vi "State Estimator.vi"(0 "Error In":errorcluster, 1 "State Estimate In":refnum<data-value>, 5 "Matrix":T2, 7 "Configuration":T1={"Accelerometer Bias"={"X (m/s)"=0.0, "Y (m/s)"=0.0, "Z (m/s)"=0.0}, "Gyroscope Bias"={"X (m/s)"=0.0, "Y (m/s)"=0.0, "Z (m/s)"=0.0}, "Steering Motor Gear Ratio"=111.0, "Steering Pully Gear Ratio"=1.0, "Steering Encoder CPR"=500.0, "Steering Motor Max RPM"=4000.0, "Wheelbase (m)"=1.12, "Fork Angle (rad)"=1.3, "Balancing Controller"={"Kp (/s)"=1.3, "Kd (1)"=3.0}, "Max Allowed Steering Angle (rad)"=0.7, "Task Periods"={"Emergency Stop (us)"=10000, "IMU (us)"=10000, "Steering Motor Encoder (us)"=10000, "State Estimator (us)"=10000, "Balancing Controller (us)"=10000, "GNSS (us)"=10000, "Logging (us)"=50000, "Drive Motor (us)"=100000, "Visualization (us)"=100000}, "Drive Motor Gear Ratio"=250.0, "lr"=0.4964, "lf"=0.5986, "lambda"=1.2217, "k1"=0.004472, "k2"=0.09678, "e1_max"=11.331, "Ad_t"=0.95971, "Bd_t"=0.01, "C_t"=2.20588, "D_t"=0.0, "Wheel radius"=0.311}, 9 "Iteration":dbl, 11 "Measurement In":refnum<data-value>, 12 "Balancing controller In":refnum<data-value>) -> (4 "Error out":errorcluster, 15 "Measurement Out":refnum<data-value>)   [LabVIEW 2021]
uses:
  Measurements.ctl
  IMU/IMU Data.ctl
  Steering Motor Encoder/Steering Motor Encoder Data.ctl
  GNSS/GNSS Data.ctl
  Logging/Controller Data.ctl
  Drive Motor/Drive Motor Data.ctl
  Steering Motor/Steering Motor Data.ctl
  State Estimate.ctl
  Configuration/Configuration.ctl
panel:
  out "Flag GPS":dbl
  out "State Estimate Out":refnum<data-value>
  out "data value":T3
  out "output cluster":T6 {"Y (m)" format="%#_10g"; "X (m)" format="%#_10g"}
  out "Balancing controller Out":refnum<data-value>
  in  "path in":path=path "libkalman_filter.so"
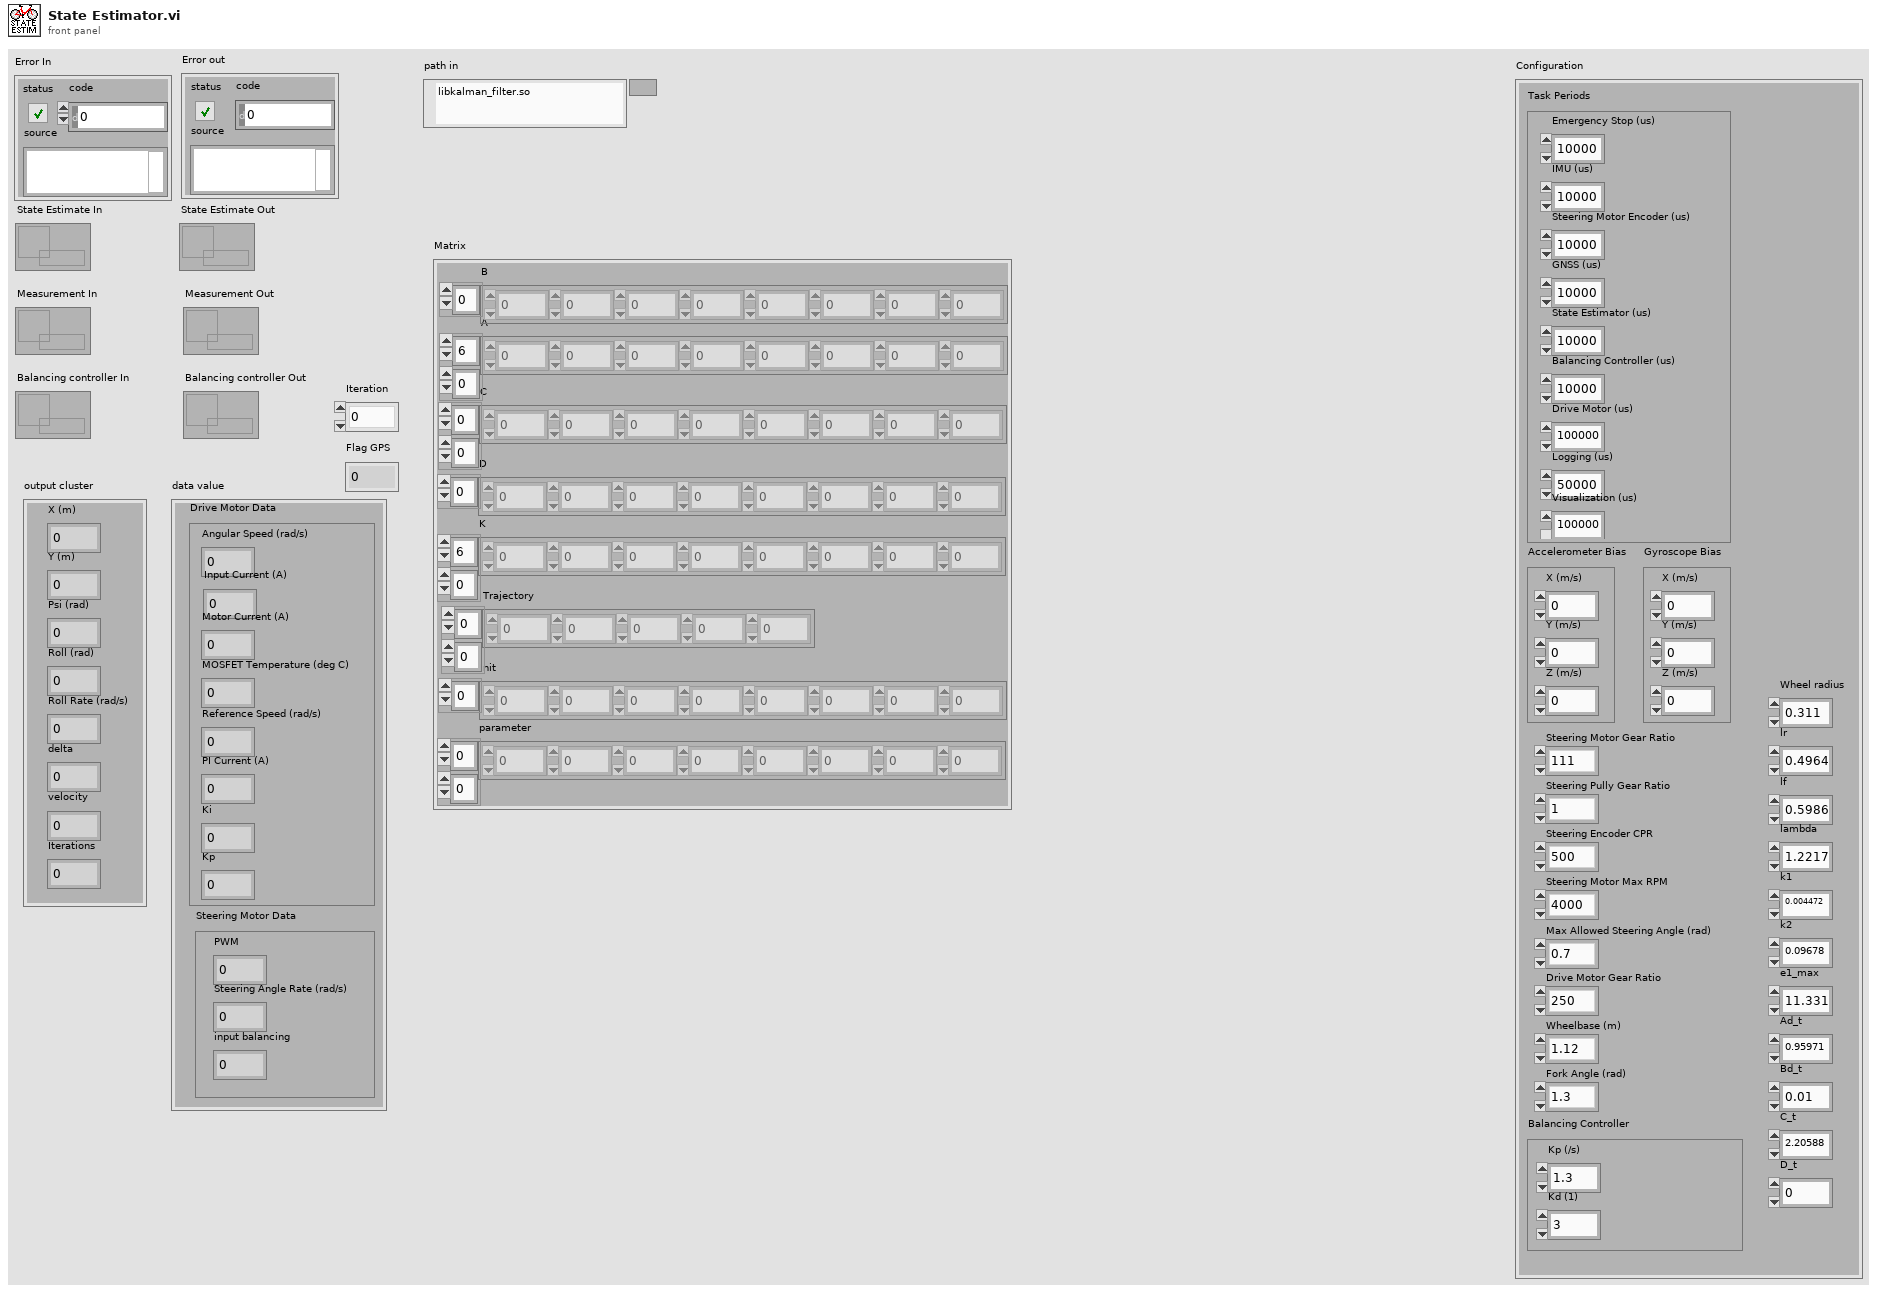
[diagram p1: front panel]
types:
  T1 = typedef "Configuration.ctl" = cluster{"Accelerometer Bias":cluster{"X (m/s)":dbl, "Y (m/s)":dbl, "Z (m/s)":dbl}, "Gyroscope Bias":cluster{"X (m/s)":dbl, "Y (m/s)":dbl, "Z (m/s)":dbl}, "Steering Motor Gear Ratio":dbl, "Steering Pully Gear Ratio":dbl, "Steering Encoder CPR":dbl, "Steering Motor Max RPM":dbl, "Wheelbase (m)":dbl, "Fork Angle (rad)":dbl, "Balancing Controller":cluster{"Kp (/s)":dbl, "Kd (1)":dbl}, "Max Allowed Steering Angle (rad)":dbl, "Task Periods":cluster{"Emergency Stop (us)":i64, "IMU (us)":i64, "Steering Motor Encoder (us)":i64, "State Estimator (us)":i64, "Balancing Controller (us)":i64, "GNSS (us)":i64, "Logging (us)":i64, "Drive Motor (us)":i64, "Visualization (us)":i64}, "Drive Motor Gear Ratio":dbl, "lr":dbl, "lf":dbl, "lambda":dbl, "k1":dbl, "k2":dbl, "e1_max":dbl, "Ad_t":dbl, "Bd_t":dbl, "C_t":dbl, "D_t":dbl, "Wheel radius":dbl}
  T2 = cluster{"B":dbl[], "A":dbl[][], "C":dbl[][], "D":dbl[], "K":dbl[][], "Trajectory":dbl[][], "Init":dbl[], "parameter":dbl[][]}
  T3 = typedef "Controller Data.ctl" = cluster{"Drive Motor Data":T4, "Steering Motor Data":T5}
  T4 = typedef "Drive Motor Data.ctl" = cluster{"Angular Speed (rad/s)":dbl, "Input Current (A)":dbl, "Motor Current (A)":dbl, "MOSFET Temperature (deg C)":dbl, "Reference Speed (rad/s)":dbl, "PI Current (A)":dbl, "Ki":dbl, "Kp":dbl}
  T5 = typedef "Steering Motor Data.ctl" = cluster{"PWM":dbl, "Steering Angle Rate (rad/s)":dbl, "input balancing":dbl}
  T6 = typedef "State Estimate.ctl" = cluster{"X (m)":dbl, "Y (m)":dbl, "Psi (rad)":dbl, "Roll (rad)":dbl, "Roll Rate (rad/s)":dbl, "delta":dbl, "velocity":dbl, "Iterations":dbl}
  T7 = typedef "Measurements.ctl" = cluster{"IMU Data":T8, "Steering Motor Encoder Data":T9, "GNSS Data":T10}
  T8 = typedef "IMU Data.ctl" = cluster{"Gyroscope":cluster{"X (rad/s)":dbl, "Y (rad/s)":dbl, "Z (rad/s)":dbl}, "Accelerometer":cluster{"X (m/s^2)":dbl, "Y (m/s^2)":dbl, "Z (m/s^2)":dbl}, "Flag IMU":dbl}
  T9 = typedef "Steering Motor Encoder Data.ctl" = cluster{"Encoder Position (counts)":i32, "Steering Angle (rad)":dbl, "Flag Steering Encoder":dbl}
  T10 = typedef "GNSS Data.ctl" = cluster{"Latitude (rad)":dbl, "Longitude (rad)":dbl, "Altitude (m)":dbl, "Speed (m/s)":dbl, "Heading (rad)":dbl, "Fix Quality":i32, "Number of Satellites":i32, "Latitude (deg)":dbl, "Longitude (deg)":dbl, "Flag GNSS":dbl}
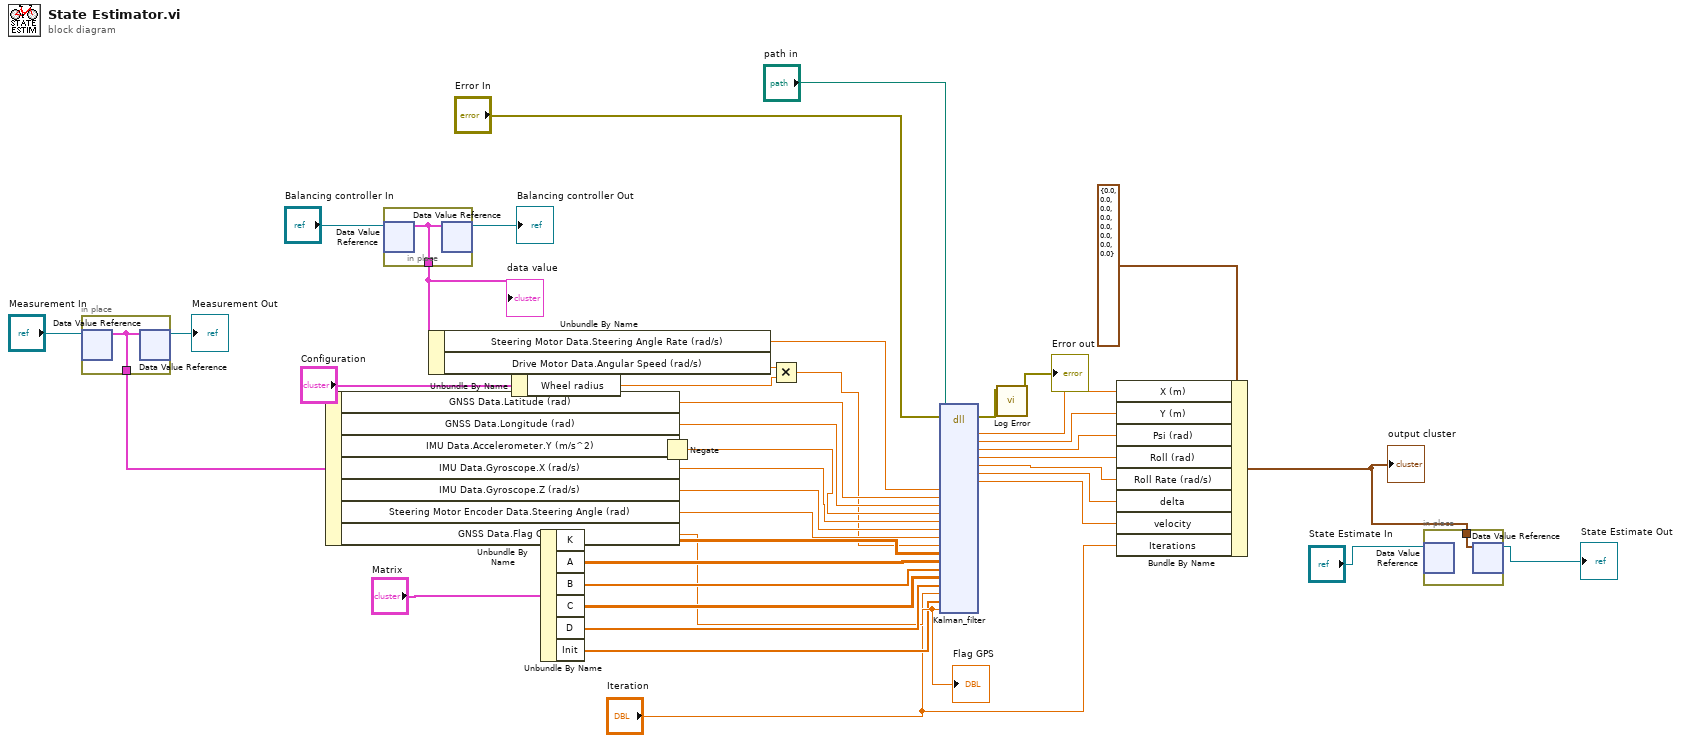
[diagram p0: block diagram]
diagram:
  n1 = in-place {
    in-place-border: [w43] -> w34
    n2 = in-place-dvr #1("Measurement In") -> (w43:T7)  [unwired: 1 out]
    n3 = in-place-dvr #1(w43) -> (→"Measurement Out":refnum<data-value>)  [unwired: 1 out]
  }
  n4 = Unbundle By Name(w34) -> ("GNSS Data.Latitude (rad)"=w22:dbl, "GNSS Data.Longitude (rad)"=w21:dbl, "IMU Data.Accelerometer.Y (m/s^2)"=w11:dbl, "IMU Data.Gyroscope.X (rad/s)"=w3:dbl, "IMU Data.Gyroscope.Z (rad/s)"=w19:dbl, "Steering Motor Encoder Data.Steering Angle (rad)"=w20:dbl, "GNSS Data.Flag GNSS"=w23:dbl)
  "Flag GPS" <- w23
  n5 = in-place {
    in-place-border: [w44] -> w33
    n6 = in-place-dvr #2("Balancing controller In") -> (w44:T3)  [unwired: 1 out]
    n7 = in-place-dvr #2(w44) -> (→"Balancing controller Out":refnum<data-value>)  [unwired: 1 out]
  }
  "data value" <- w33
  n8 = Unbundle By Name(w33) -> ("Steering Motor Data.Steering Angle Rate (rad/s)"=w9:dbl, "Drive Motor Data.Angular Speed (rad/s)"=w12:dbl)
  n9 = Unbundle By Name("Configuration") -> ("Wheel radius"=w4:dbl)
  n10 = Unbundle By Name("Matrix") -> ("K"=w28:dbl[][], "A"=w27:dbl[][], "B"=w26:dbl[], "C"=w25:dbl[][], "D"=w24:dbl[], "Init"=w13:dbl[])
  n11 = Negate(x=w11) -> (-x=w10:dbl)
  n12 = Multiply(x=w12, y=w4) -> (x*y=w2:dbl)
  n13 = dll-call lib="libkalman_filter.so" fn="Kalman_filter"(path in="path in", error in="Error In", "dotdelta"=w9, "latitude"=w22, "longitude"=w21, "a_y"=w10, "w_x"=w3, "w_z"=w19, "delta_enc"=w20, "speed"=w2, "Kalman_Gain"=w28, "A_d"=w27, "B_d"=w26, "C"=w25, "D"=w24, "Reset"="Iteration", "init"=w13, "GPSflag"=w23) -> (error out=w29:errorcluster, "X"=w18:dbl, "Y"=w17:dbl, "Psi"=w16:dbl, "roll"=w8:dbl, "rollRate"=w7:dbl, "delta"=w15:dbl, "v"=w14:dbl)  [unwired: 25 in, 1 out]
  n14 = call "Log Error.vi"("Error In"=w29) -> ("Error Out"=→"Error out":errorcluster)  [unwired: 10 in]
  n15 = Bundle By Name(cluster=T6 {"X (m)"=0.0, "Y (m)"=0.0, "Psi (rad)"=0.0, "Roll (rad)"=0.0, "Roll Rate (rad/s)"=0.0, "delta"=0.0, "velocity"=0.0, "Iterations"=0.0} ("State Estimate"), "X (m)"=w18, "Y (m)"=w17, "Psi (rad)"=w16, "Roll (rad)"=w8, "Roll Rate (rad/s)"=w7, "delta"=w15, "velocity"=w14, "Iterations"="Iteration") -> (w30:T6)
  "output cluster" <- w30
  n16 = in-place {
    in-place-border: w30 -> [w45]
    n17 = in-place-dvr #3("State Estimate In") -> ()  [unwired: 2 out]
    n18 = in-place-dvr #3(w45) -> (→"State Estimate Out":refnum<data-value>)  [unwired: 1 out]
  }
